vi "AIT 664 - Read Output VL XML.vi"(0 "Node Reg":refnum<k20>, 11 "error in (no error)":errorcluster) -> (4 "Output VL":T1, 15 "error out":errorcluster)   [LabVIEW 2013, in "AIT 664 Custom Device.lvlib"]
doc: "Read in Output VL XML"
uses:
  AIT 664 Custom Device.lvlib
  Controls/664 - XML Output VL.ctl
  Controls/664 - XML Tx Message Port.ctl
  Controls/664 - Sampling Type.ctl
  Controls/664 -Param.ctl
  <vilib>/xml/Close Reference(NNMap).vi
  <vilib>/xml/Close Reference(Node).vi
  <resource>/objmgr/DOMUserDefRef.rc
  <vilib>/xml/NI_XML.lvlib
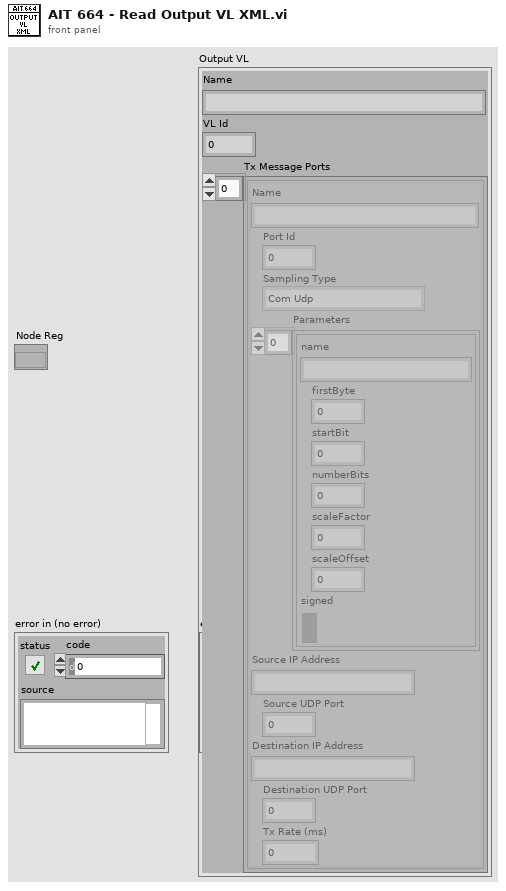
[diagram p1: front panel]
types:
  T1 = typedef "AIT 664 Custom Device.lvlib/664 - XML Output VL.ctl" = cluster{"Name":string, "VL Id":u32, "Tx Message Ports":T2[]}
  T2 = typedef "AIT 664 Custom Device.lvlib/664 - XML Tx Message Port.ctl" = cluster{"Name":string, "Port Id":u32, "Sampling Type":T3, "Parameters":T4[], "Source IP Address":string, "Source UDP Port":u32, "Destination IP Address":string, "Destination UDP Port":u32, "Tx Rate (ms)":u32}
  T3 = typedef "AIT 664 Custom Device.lvlib/664 - Sampling Type.ctl" = enum16{"Com Udp", "Com Udp Queuing", "Sap Udp", "Sap Ip", "Sap Mac", "Unknown"}
  T4 = typedef "AIT 664 Custom Device.lvlib/664 -Param.ctl" = cluster{"name":string, "firstByte":i32, "startBit":i32, "numberBits":i32, "scaleFactor":dbl, "scaleOffset":dbl, "signed":bool}
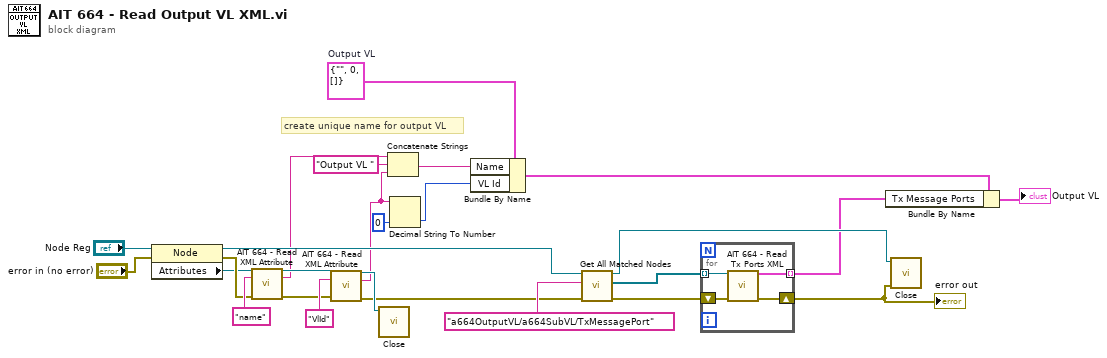
[diagram p0: block diagram]
diagram:
  w23 = T1 {"Name"="", "VL Id"=0, "Tx Message Ports"=[]}  # Output VL
  # "create unique name for output VL"
  n1 = property class="Node"(reference="Node Reg", error in="error in (no error)") -> (reference out=w13:refnum<k20>, error out=w18:errorcluster, "Attributes"=w16:refnum<k20>)
  n2 = call "AIT 664 - Read XML Attribute.vi"("Attributes In"=w16, "Attribute Name"="name", "error in (no error)"=w18) -> ("Attributes Out"=w21:refnum<k20>, "Attribute Text"=w2:string, "error out"=w20:errorcluster)  [unwired: 10 in]
  n3 = call "AIT 664 - Read XML Attribute.vi"("Attributes In"=w21, "Attribute Name"="VlId", "error in (no error)"=w20) -> ("Attributes Out"=w26:refnum<k20>, "Attribute Text"=w3:string, "error out"=w12:errorcluster)  [unwired: 10 in]
  n4 = call-poly <vilib>:"Close.vi"("named node map"=w26) -> ()  [unwired: 8 in, 1 out]
  n5 = Concatenate Strings(w2, "Output VL " ("string"), w3) -> (w1:string)
  n6 = Decimal String To Number(string=w3, default (0L)=u32 0 ("default (0 I32)")) -> (number=w25:u32)  [unwired: 1 in, 1 out]
  n7 = Bundle By Name(cluster=w23, "Name"=w1, "VL Id"=w25) -> (w6:T1)
  n8 = call <vilib>:"Get All Matched Nodes.vi"("error in (no error)"=w12, "XPath expression"="a664OutputVL/a664SubVL/TxMessagePort", "node in"=w13) -> ("error out"=w10:errorcluster, "node result array"=w11:refnum<k20>[], "node out"=w8:refnum<k20>)  [unwired: 6 in]
  n9 = for {
    tunnel: w11 -> [w30] mode=indexing
    shift-right: [w27] -> w9
    shift-left: w10 -> [w29]
    tunnel: [w28] -> w5 mode=indexing
    n10 = call "AIT 664 - Read Tx Ports XML.vi"("Refnum in"=w30, "error in (no error)"=w29) -> ("Tx Message Port"=w28:T2, "error out"=w27:errorcluster)  [unwired: 12 in]
  }
  "error out" <- w9
  n11 = Bundle By Name(cluster=w6, "Tx Message Ports"=w5) -> (→"Output VL":T1)
  n12 = call-poly <vilib>:"Close.vi"("error in (no error)"=w9, "node"=w8) -> ()  [unwired: 7 in, 1 out]
